vi "SimpleLiveAppStreamSaving.vi"() -> ()   [LabVIEW 2020]
uses:
  C:/Users/Public/Documents/Photometrics/PMQI-LabViewSamples/Examples/2018/Dependencies/PVCamNET.dll
  Dependencies/PVCamNET.dll
panel:
  out "Multi Page TIFF Size Read":u64 max=1 step=1
  in  "Multi Page TIFF Size [bytes]":u64 max=1 step=1
  out "Big TIFF":bool
  in  "BigTIFF On/Off":bool
  out "Available Ram":u64
  out "Disk Stream Queue Size":u64
  out "Dropped Frames":i32
  out "Buffer Index":i32
  in  "Path":path
  out "StreamSavingPath":string
  in  "File format":u8 max=1 step=1
  out "Stream Saving":bool
  out "Display":bool
  in  "Stream Saving On/Off":bool
  in  "Display On/Off":bool
  in  "Exposure Time [ms]":dbl
  in  "Live":bool
  in  "Camera Status":bool
  in  "Uninit":bool
  in  "Live stop":bool
  in  "Live start":bool
  in  "Init":bool
  # "SimpleLiveAppStreamSaving.vi\n\nDescription:\nThis sample code lets the user use stream saving with live mode in an event driven structure.\n\nSteps to run:\n1. Click \"Run\"\n2. Click \"Open\"\n3. Enter Exposure Time\n4. Turn On/Off display\n5. Set \"0\" to Format ( Raw=0 Tiff =1)\n6. Toggle Big TIFF\n7. Enter multi page TIFF size (at default the staxk size is 2GB for regular TIFF and 4GB for Big TIFF)\n8. Select the path for images to be saved at\n9. Turn \"On\" Stream Saving\n10. Click \"Live start\"\n11. Click \"Live stop\"\n12. Click \"Close\""
  # "Note about Tiff and BigTiff saving:\n\n\tAt default images are stored with regular Tiff and the maximum multi-image size is 2GB.\n\nIf you would like to save 6GB with Big Tiff then\n    BIG TIFF ON /OFF = ON;\n    Multi Page TIFF Size = 6442450944; (in bytes)\n\t\t\nIfyou would like to save 1 page per file with regular Tiff\n    BIG TIFF ON /OFF = ON;\n    Multi Page TIFF Size =1; (any number smaller than a frame size except 0)\n\t\t\nIf you would like to save 2GB with regular Tiff then\n    BIG TIFF ON /OFF = OFF;\n    Multi Page TIFF Size = 2147483648;"
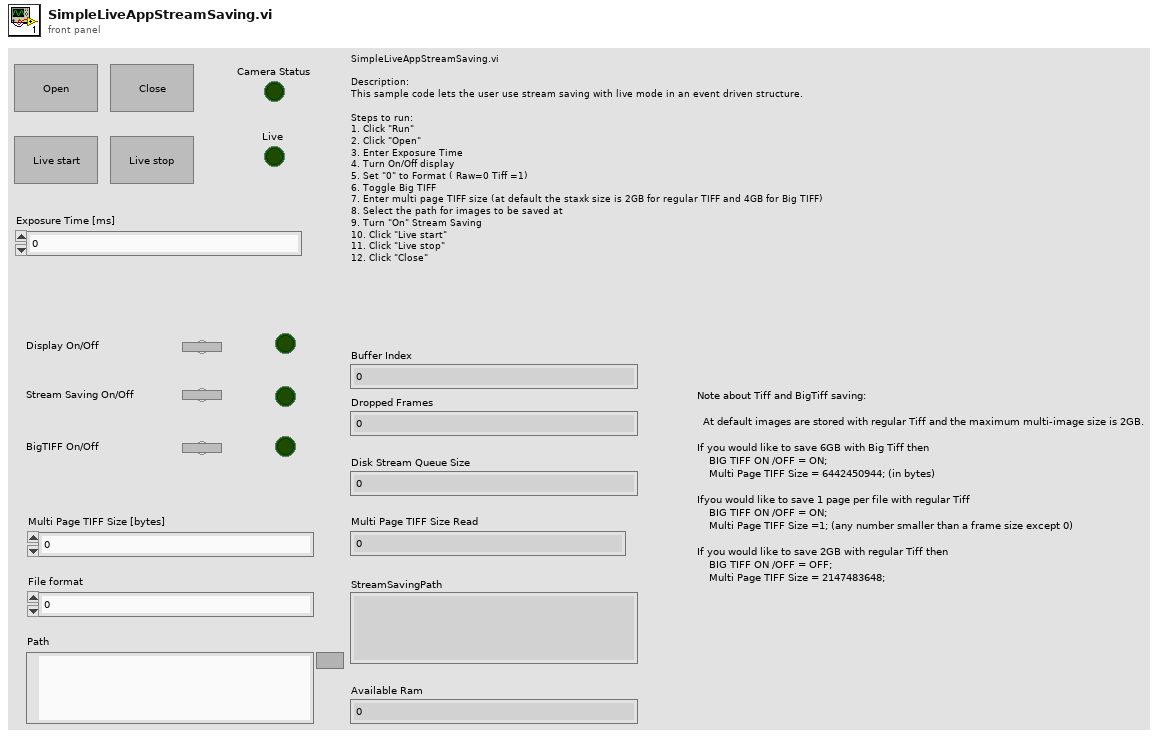
[diagram p1: front panel]
types:
  T1 = cluster{"Buffer Index":refnum<vi>, "Dropped Frames":refnum<vi>, "Disk Stream Queue Size":refnum<vi>, "Available Ram":refnum<vi>}
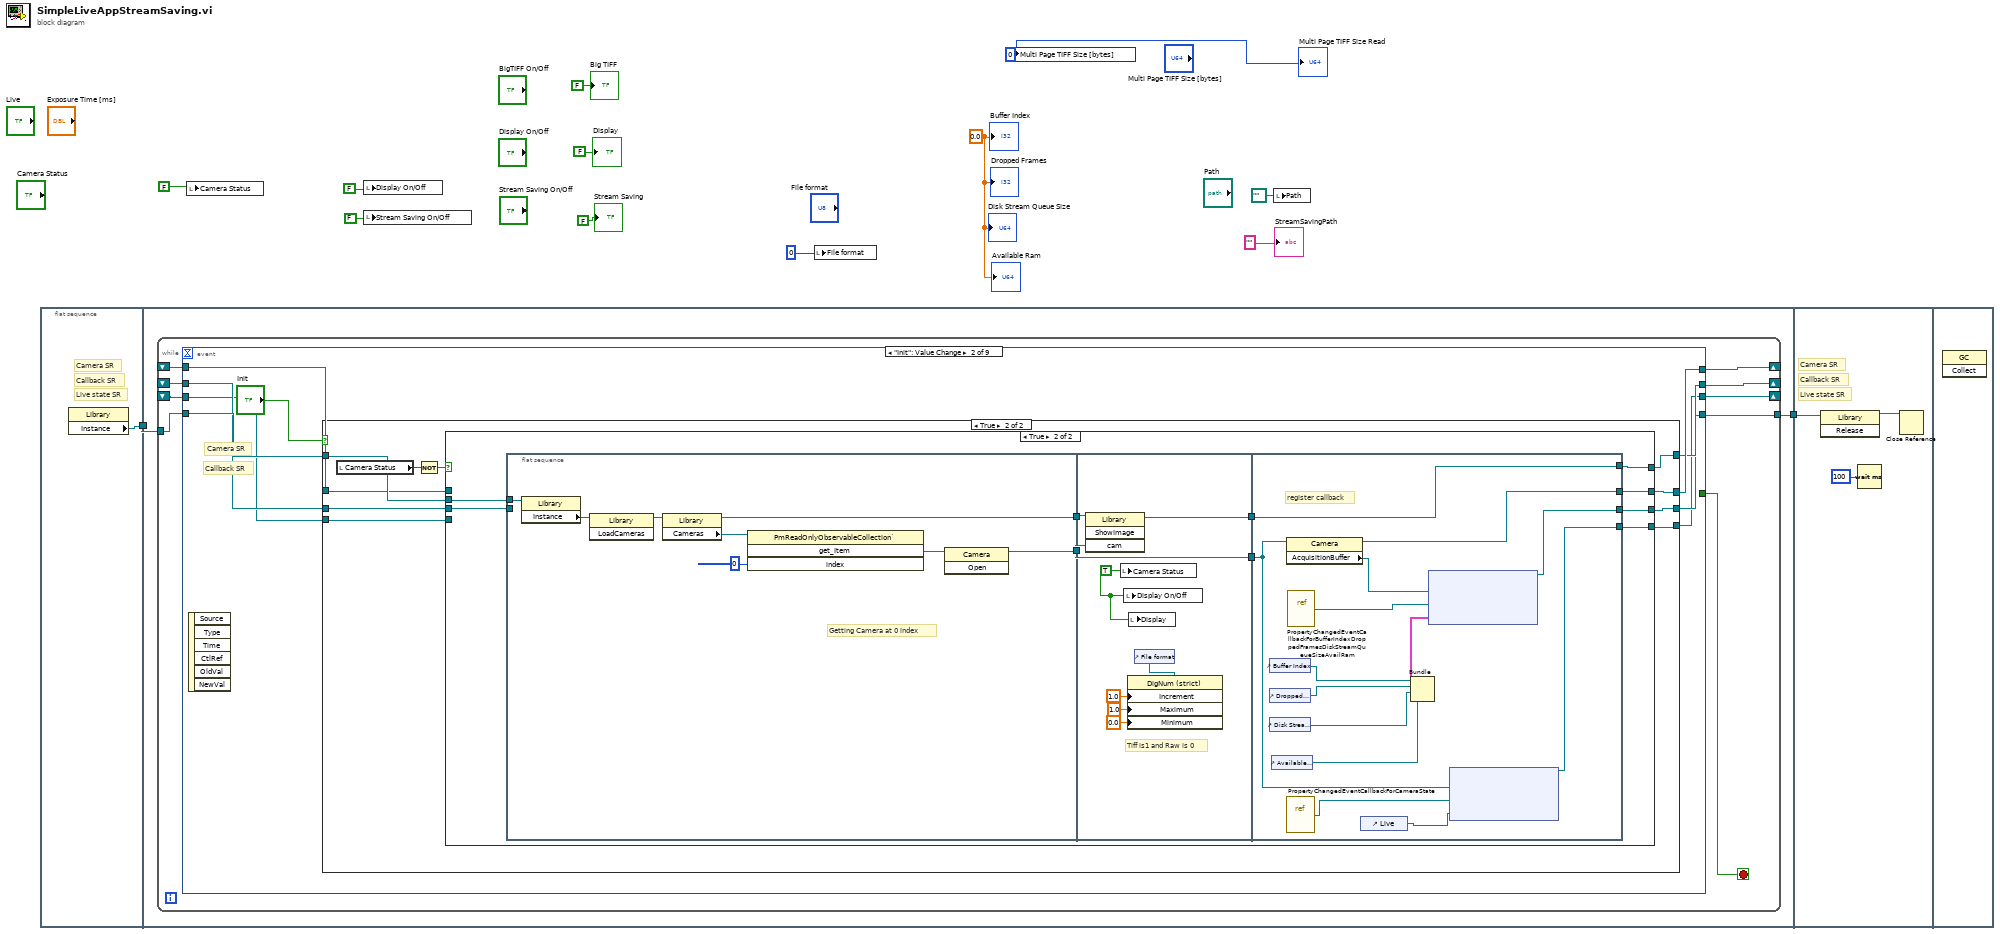
[diagram p0: block diagram]
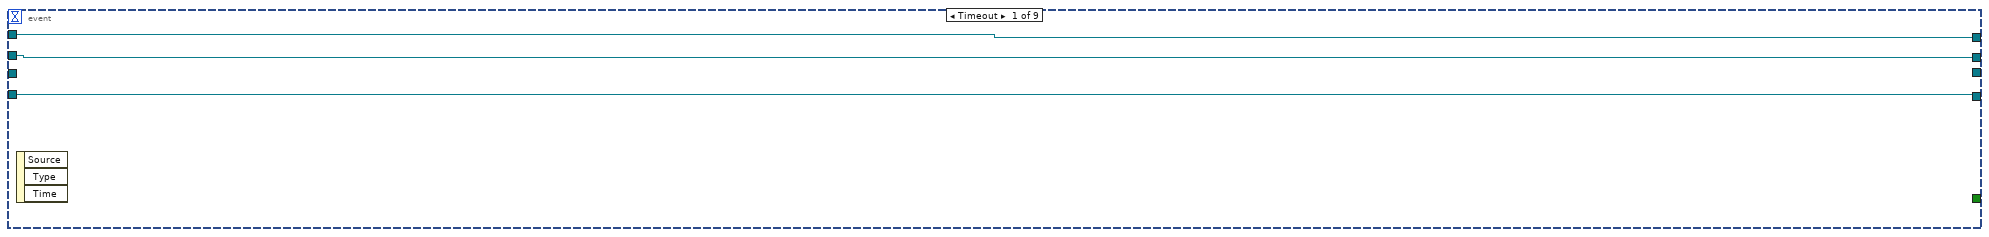
[diagram p2: hidden frame]
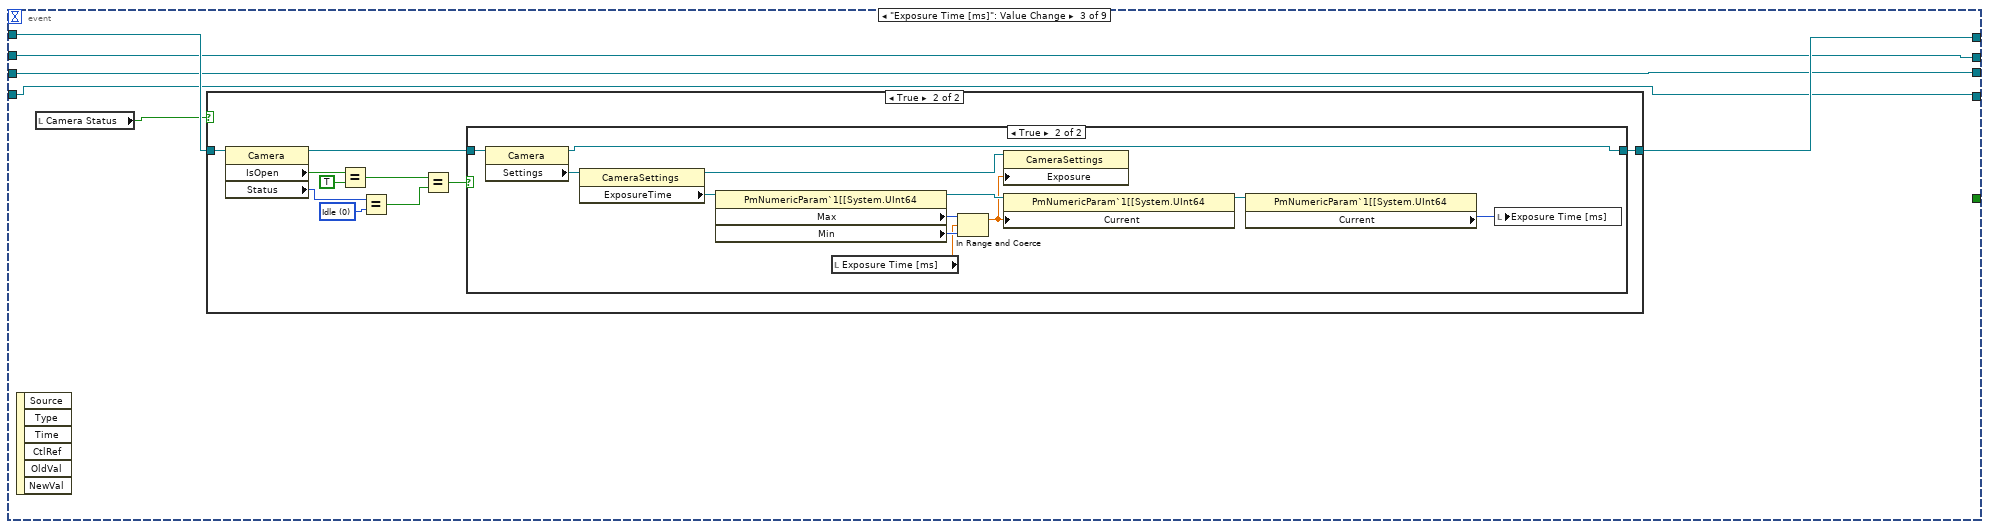
[diagram p5: hidden frame]
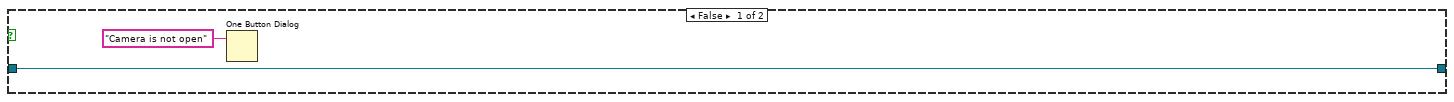
[diagram p6: hidden frame]
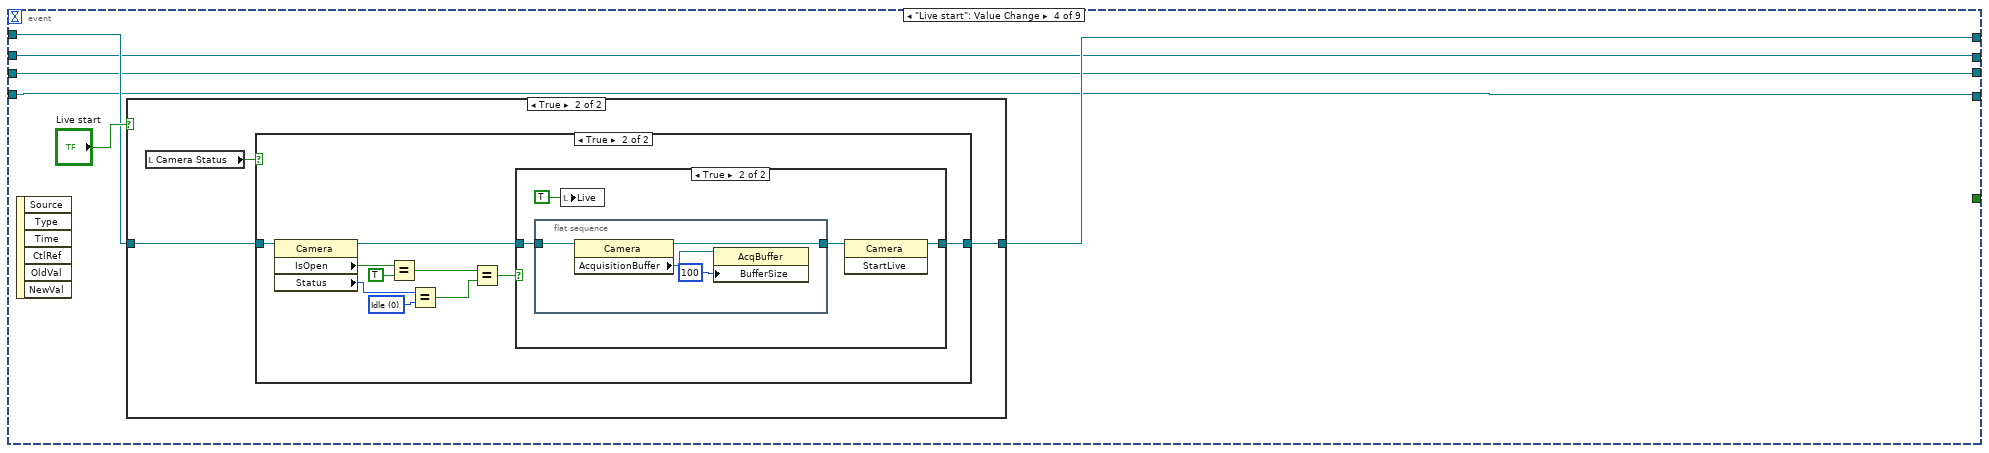
[diagram p8: hidden frame]
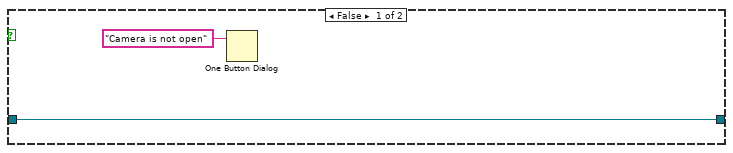
[diagram p10: hidden frame]
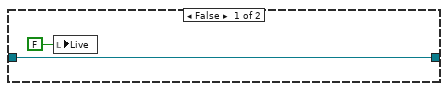
[diagram p11: hidden frame]
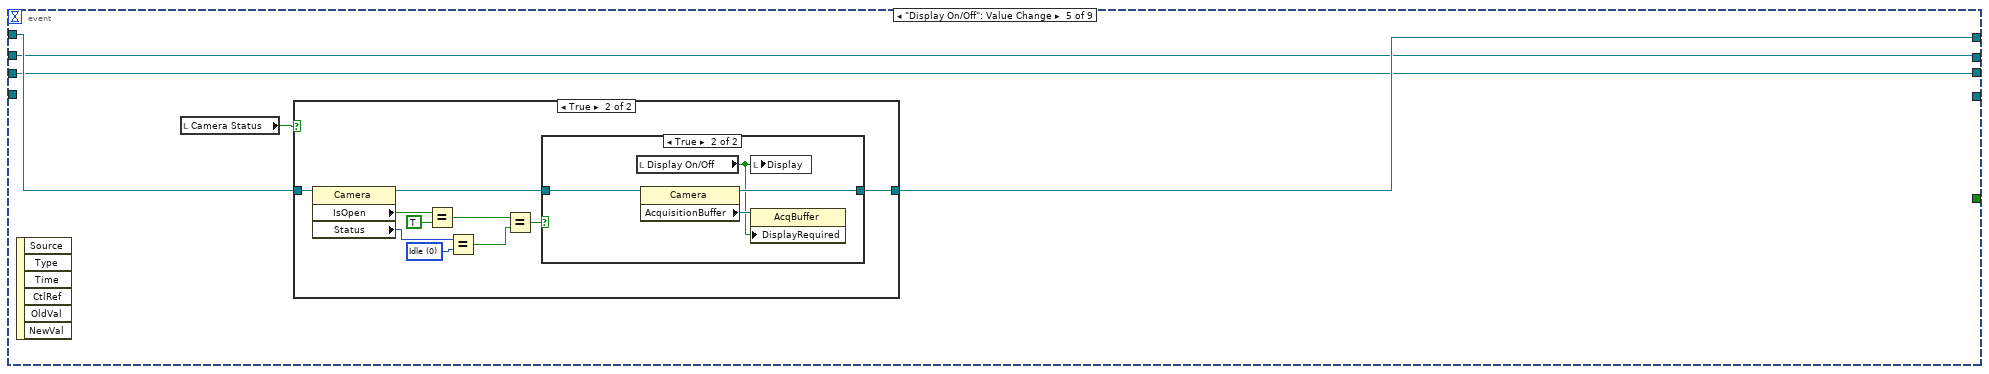
[diagram p12: hidden frame]
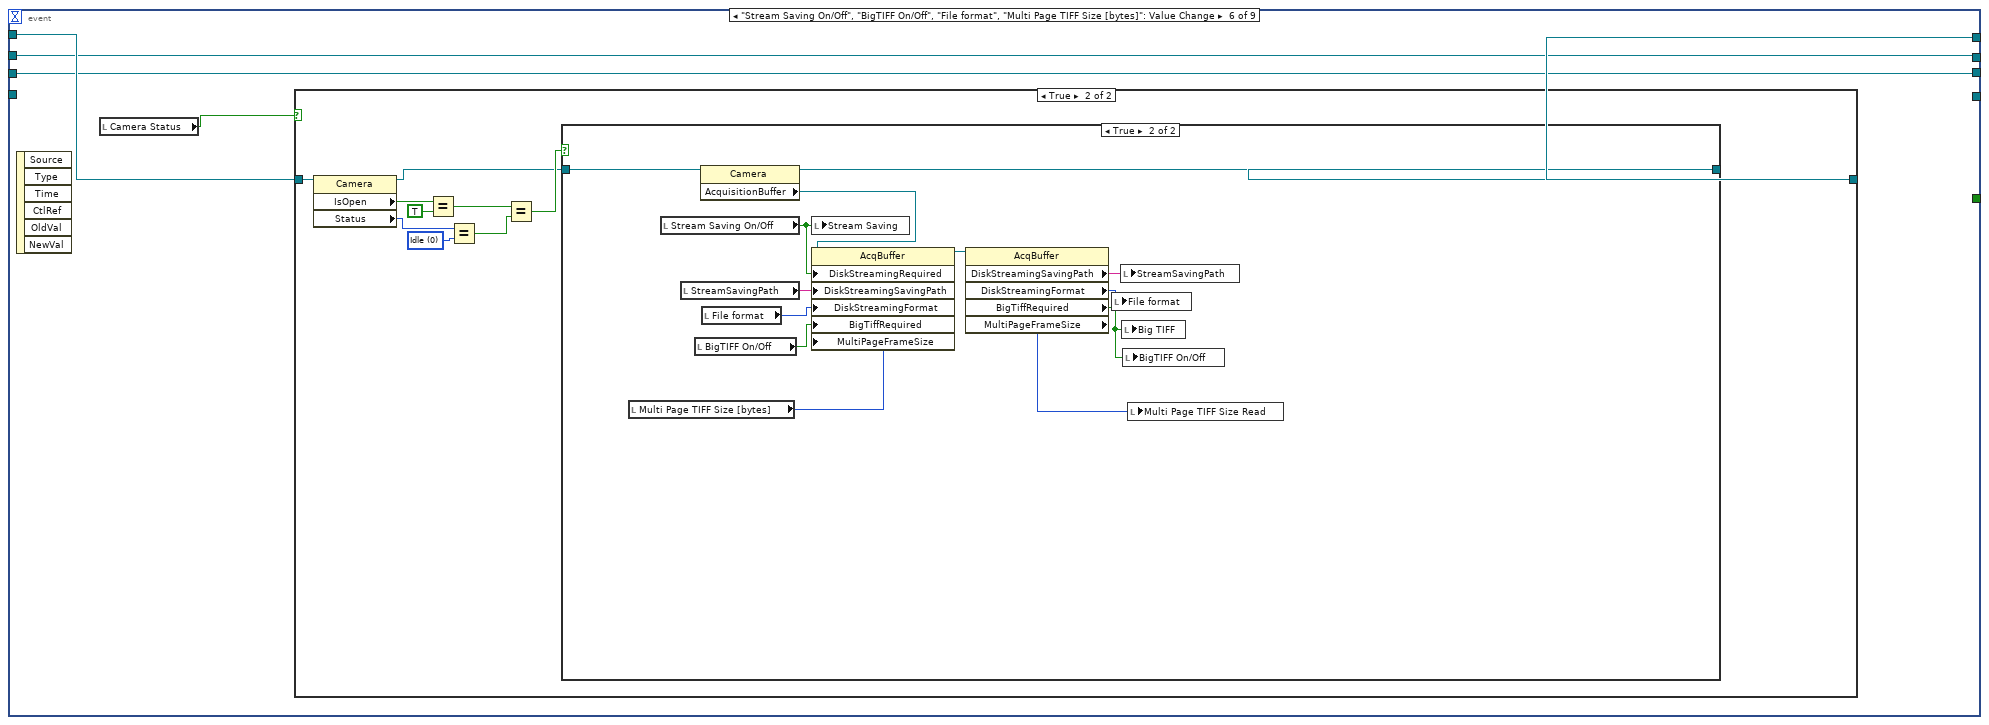
[diagram p15: hidden frame]
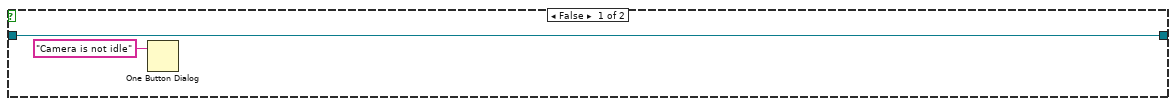
[diagram p17: hidden frame]
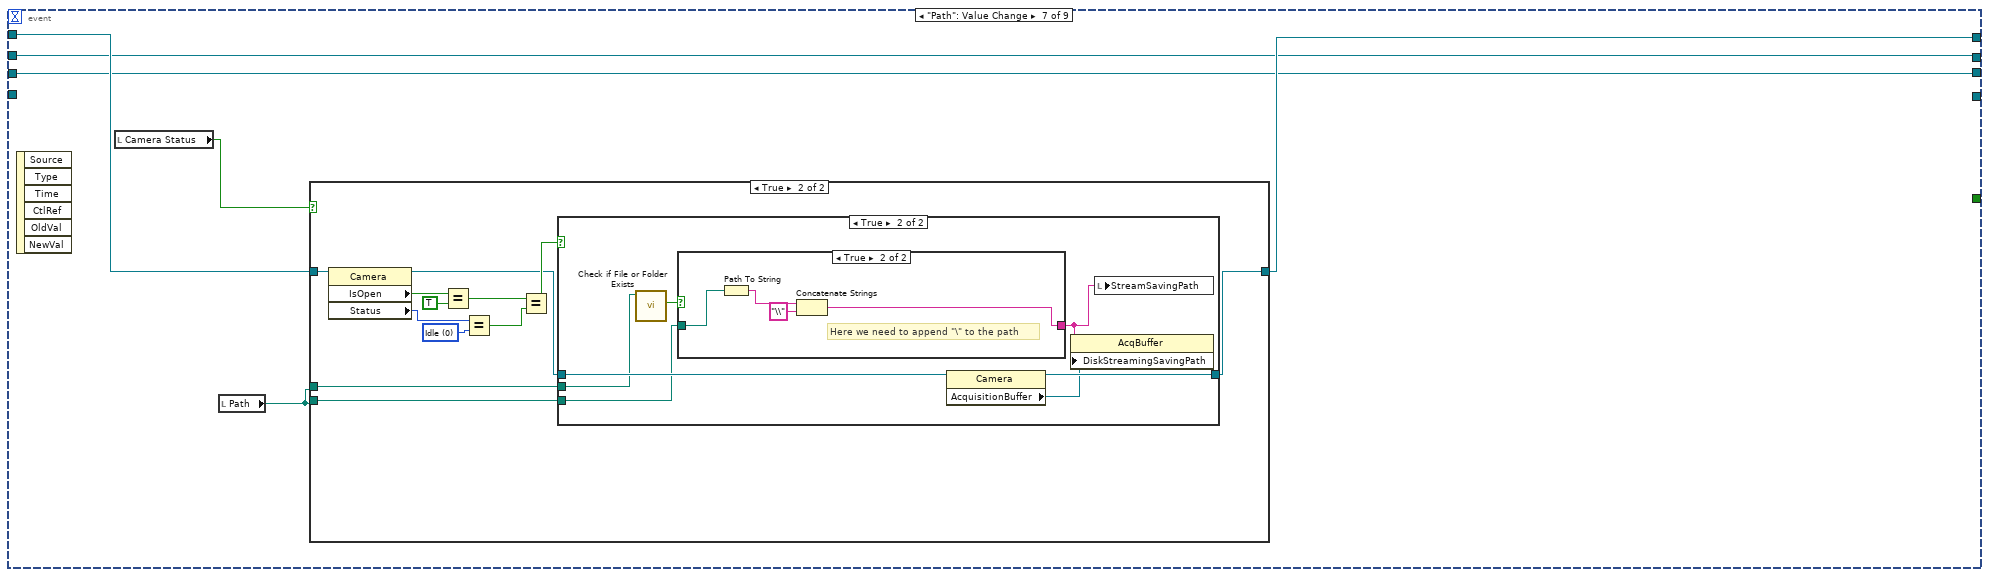
[diagram p18: hidden frame]
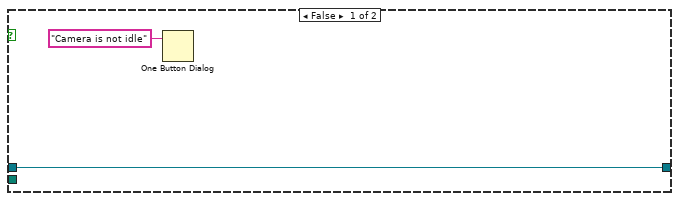
[diagram p20: hidden frame]
diagram:
  w1 = u8 0 ("Multi Page Tiff Size")
  w3 = 0.0 ("Buffer Index")
  n1 = flat-sequence {
    tunnel: [w14] -> w13
    tunnel: w13 -> [w16]
    tunnel: [w15] -> w12
    tunnel: w12 -> [w327]
    frame #0 {
      # "Live state SR"
      # "Callback SR"
      # "Camera SR"
      n2 = property class="Library"() -> ("Instance"=w14:refnum<k24>)  [unwired: 2 in, 2 out]
    }
    frame #1 {
      n3 = while {
        tunnel: w16 -> [w25]
        shift-right: [w24] -> _
        shift-left: _ -> [w22]
        tunnel: [w23] -> w15
        shift-right: [w20] -> _
        shift-left: _ -> [w19]
        shift-right: [w18] -> _
        shift-left: _ -> [w17]
        stop <- w21 stop-if-true
        n4 = event shown="[1] \"Init\": Value Change" {
          selector: _ -> [_ _ _ _ _ _ _ _ _]
          dyn-events: _ -> [_ _ _ _ _ _ _ _ _]
          timeout: _ -> [_ _ _ _ _ _ _ _ _]
          tunnel: w25 -> [w26 w37 w98 w129 _ _ _ _ w277]
          tunnel: [w27 w36 w100 w130 w162 w182 w214 w248 w278] -> w24
          tunnel: [w26 w35 w98 w129 _ _ _ _ w277] -> w23
          tunnel: w22 -> [w27 w34 w101 w131 w163 w183 w215 w249 w272]
          tunnel: [_ _ _ _ _ _ _ _ w276] -> w21
          tunnel: [w28 w32 w97 w127 w160 w181 w213 w247 w273] -> w20
          tunnel: w19 -> [w28 w31 w97 w127 w160 w181 w213 w247 w274]
          tunnel: [_ w30 w96 w128 w159 w180 w212 w245 w271] -> w18
          tunnel: w17 -> [_ w29 w96 w128 w159 w180 w212 w245 w270]
          event Timeout {
            n5 = event-data() -> ()  [unwired: 1 in, 3 out]
          }
          event "Init": Value Change {
            # "Camera SR"
            # "Callback SR"
            n6 = event-data() -> ()  [unwired: 1 in, 6 out]
            n7 = case shown="True" "Init" {
              tunnel: w37 -> [w41 w51]
              tunnel: [w40 w50] -> w36
              tunnel: [w41 w44] -> w35
              tunnel: w34 -> [w40 w47]
              tunnel: [w39 w45] -> w32
              tunnel: w31 -> [w39 w46]
              tunnel: [w38 w43] -> w30
              tunnel: w29 -> [w38 w42]
              frame False {
              }
              frame True {
                n8 = local read "Camera Status"() -> (w49:bool)
                n9 = Not(x=w49) -> (.not. x?=w48:bool)
                n10 = case shown="True" w48 {
                  tunnel: w51 -> [w54 w63]
                  tunnel: [w55 w62] -> w50
                  tunnel: [w54 w61] -> w44
                  tunnel: w47 -> [w55 _]
                  tunnel: [w53 w58] -> w45
                  tunnel: w46 -> [w53 w57]
                  tunnel: [w52 w56] -> w43
                  tunnel: w42 -> [w52 _]
                  frame False {
                  }
                  frame True {
                    n11 = flat-sequence {
                      tunnel: w63 -> [w68]
                      tunnel: [w70] -> w65
                      tunnel: [w69] -> w64
                      tunnel: w57 -> [_]
                      tunnel: w65 -> [w80]
                      tunnel: w64 -> [w81]
                      tunnel: [w81] -> w60
                      tunnel: [w79] -> w59
                      tunnel: [w95] -> w61
                      tunnel: [w89] -> w62
                      tunnel: w60 -> [w88]
                      tunnel: w59 -> [w95]
                      tunnel: [w84] -> w58
                      tunnel: [w85] -> w56
                      frame #0 {
                        # "Getting Camera at 0 index"
                        n12 = property class="Library"(reference=w68) -> ("Instance"=w67:refnum<k24>)  [unwired: 1 in, 2 out]
                        n13 = invoke class="Library" method="LoadCameras"(reference=w67) -> (reference out=w66:refnum<k24>)  [unwired: 2 in, 2 out]
                        n14 = property class="Library"(reference=w66) -> (reference out=w70:refnum<k24>, "Cameras"=w73:refnum<k24>)  [unwired: 1 in, 1 out]
                        n15 = invoke class="PmReadOnlyObservableCollection`" method="get_Item"(reference=w73, "index"=0) -> ("get_Item"=w71:refnum<k24>)  [unwired: 2 in, 3 out]
                        n16 = invoke class="Camera" method="Open"(reference=w71) -> (reference out=w69:refnum<k24>)  [unwired: 2 in, 2 out]
                      }
                      frame #1 {
                        w78 = TRUE ("Camera Status")
                        # "Tiff is1 and Raw is 0"
                        n17 = invoke class="Library" method="ShowImage"(reference=w80, "cam"=w81) -> (reference out=w79:refnum<k24>)  [unwired: 2 in, 3 out]
                        n18 = local write "Camera Status"(w78) -> ()
                        n19 = local write "Display On/Off"(w78) -> ()
                        n20 = local write "Display"(w78) -> ()
                        n21 = control-ref of="File format"() -> (w77:refnum<vi>)
                        n22 = property class="DigNum (strict)"(reference=w77, "Increment"=1.0 ("Data Entry Limits:Increment"), "Maximum"=1.0 ("Data Entry Limits:Maximum"), "Minimum"=0.0 ("Data Entry Limits:Minimum")) -> ()  [unwired: 1 in, 2 out]
                      }
                      frame #2 {
                        # "register callback"
                        n23 = control-ref of="Buffer Index"() -> (w94:refnum<vi>)
                        n24 = control-ref of="Dropped Frames"() -> (w93:refnum<vi>)
                        n25 = control-ref of="Disk Stream Queue Size"() -> (w92:refnum<vi>)
                        n26 = control-ref of="Available Ram"() -> (w83:refnum<vi>)
                        n27 = property class="Camera"(reference=w88) -> (reference out=w89:refnum<k24>, "AcquisitionBuffer"=w90:refnum<k24>)  [unwired: 1 in, 1 out]
                        n28 = vi-ref "PropertyChangedEventCallbackForCameraState.vi"() -> ("vi reference"=w87:refnum<vi>)
                        n29 = vi-ref "PropertyChangedEventCallbackForBufferIndexDroppedFramesDiskStreamQueueSizeAvailRam.vi"() -> ("vi reference"=w82:refnum<vi>)
                        n30 = control-ref of="Live"() -> (w86:refnum<vi>)
                        n31 = Bundle("Buffer Index"=w94, "Dropped Frames"=w93, "Disk Stream Queue Size"=w92, "Available Ram"=w83) -> (w91:T1)  [unwired: 1 in]
                        n32 = node(w90, w82, w91) -> (w84:refnum<k27>)  [unwired: 2 in, 1 out]
                        n33 = node(w88, w87, w86) -> (w85:refnum<k27>)  [unwired: 2 in, 1 out]
                      }
                    }
                  }
                }
              }
            }
          }
          event "Exposure Time [ms]": Value Change {
            n34 = event-data() -> ()  [unwired: 1 in, 6 out]
            n35 = local read "Camera Status"() -> (w99:bool)
            n36 = case shown="True" w99 {
              tunnel: w101 -> [w103 w107]
              tunnel: [w103 w104] -> w100
              frame False {
                n37 = One Button Dialog(message="Camera is not open") -> ()  [unwired: 1 in, 1 out]
              }
              frame True {
                w112 = 0 items=["Idle", "Capturing"] ("Status")
                n38 = property class="Camera"(reference=w107) -> (reference out=w105:refnum<k24>, "IsOpen"=w111:bool, "Status"=w113:i32)  [unwired: 1 in, 1 out]
                n39 = Equal?(x=w111, y=TRUE) -> (x = y?=w109:bool)
                n40 = Equal?(x=w113, y=w112) -> (x = y?=w108:bool)
                n41 = Equal?(x=w109, y=w108) -> (x = y?=w106:bool)
                n42 = case shown="True" w106 {
                  tunnel: w105 -> [w114 w126]
                  tunnel: [w114 w115] -> w104
                  frame False {
                  }
                  frame True {
                    n43 = property class="Camera"(reference=w126) -> (reference out=w115:refnum<k24>, "Settings"=w125:refnum<k24>)  [unwired: 1 in, 1 out]
                    n44 = property class="CameraSettings"(reference=w125) -> (reference out=w118:refnum<k24>, "ExposureTime"=w119:refnum<k24>)  [unwired: 1 in, 1 out]
                    n45 = property class="PmNumericParam`1[[System.UInt64"(reference=w119) -> (reference out=w122:refnum<k24>, "Max"=w124:u64, "Min"=w123:u64)  [unwired: 1 in, 1 out]
                    n46 = local read "Exposure Time [ms]"() -> (w117:dbl)
                    n47 = In Range and Coerce(upper limit=w124, x=w117, lower limit=w123) -> (coerced(x)=w120:dbl)  [unwired: 1 out]
                    n48 = property class="CameraSettings"(reference=w118, "Exposure"=w120) -> ()  [unwired: 1 in, 2 out]
                    n49 = property class="PmNumericParam`1[[System.UInt64"(reference=w122, "Current"=w120) -> (reference out=w121:refnum<k24>)  [unwired: 1 in, 1 out]
                    n50 = property class="PmNumericParam`1[[System.UInt64"(reference=w121) -> ("Current"=w116:u64)  [unwired: 1 in, 2 out]
                    n51 = local write "Exposure Time [ms]"(w116) -> ()
                  }
                }
              }
            }
          }
          event "Live start": Value Change {
            n52 = event-data() -> ()  [unwired: 1 in, 6 out]
            n53 = case shown="True" "Live start" {
              tunnel: w131 -> [w133 w136]
              tunnel: [w133 w135] -> w130
              frame False {
              }
              frame True {
                n54 = local read "Camera Status"() -> (w134:bool)
                n55 = case shown="True" w134 {
                  tunnel: w136 -> [w137 w142]
                  tunnel: [w137 w140] -> w135
                  frame False {
                    n56 = One Button Dialog(message="Camera is not open") -> ()  [unwired: 1 in, 1 out]
                  }
                  frame True {
                    w147 = 0 items=["Idle", "Capturing"] ("Status")
                    n57 = property class="Camera"(reference=w142) -> (reference out=w141:refnum<k24>, "IsOpen"=w146:bool, "Status"=w148:i32)  [unwired: 1 in, 1 out]
                    n58 = Equal?(x=w146, y=TRUE) -> (x = y?=w144:bool)
                    n59 = Equal?(x=w148, y=w147) -> (x = y?=w143:bool)
                    n60 = Equal?(x=w144, y=w143) -> (x = y?=w139:bool)
                    n61 = case shown="True" w139 {
                      tunnel: w141 -> [w150 w152]
                      tunnel: [w150 w153] -> w140
                      frame False {
                        n62 = local write "Live"(FALSE ("Live 2")) -> ()
                      }
                      frame True {
                        n63 = flat-sequence {
                          tunnel: w152 -> [w158]
                          tunnel: [w155] -> w151
                          frame #0 {
                            n64 = property class="Camera"(reference=w158) -> (reference out=w155:refnum<k24>, "AcquisitionBuffer"=w157:refnum<k24>)  [unwired: 1 in, 1 out]
                            n65 = property class="AcqBuffer"(reference=w157, "BufferSize"=100) -> ()  [unwired: 1 in, 2 out]
                          }
                        }
                        n66 = local write "Live"(TRUE ("Live")) -> ()
                        n67 = invoke class="Camera" method="StartLive"(reference=w151) -> (reference out=w153:refnum<k24>)  [unwired: 2 in, 2 out]
                      }
                    }
                  }
                }
              }
            }
          }
          event "Display On/Off": Value Change {
            n68 = event-data() -> ()  [unwired: 1 in, 6 out]
            n69 = local read "Camera Status"() -> (w161:bool)
            n70 = case shown="True" w161 {
              tunnel: w163 -> [w164 w168]
              tunnel: [w164 w165] -> w162
              frame False {
              }
              frame True {
                w173 = 0 items=["Idle", "Capturing"] ("Status")
                n71 = property class="Camera"(reference=w168) -> (reference out=w166:refnum<k24>, "IsOpen"=w172:bool, "Status"=w174:i32)  [unwired: 1 in, 1 out]
                n72 = Equal?(x=w172, y=TRUE) -> (x = y?=w170:bool)
                n73 = Equal?(x=w174, y=w173) -> (x = y?=w169:bool)
                n74 = Equal?(x=w170, y=w169) -> (x = y?=w167:bool)
                n75 = case shown="True" w167 {
                  tunnel: w166 -> [w175 w179]
                  tunnel: [w175 w177] -> w165
                  frame False {
                  }
                  frame True {
                    n76 = local read "Display On/Off"() -> (w176:bool)
                    n77 = property class="Camera"(reference=w179) -> (reference out=w177:refnum<k24>, "AcquisitionBuffer"=w178:refnum<k24>)  [unwired: 1 in, 1 out]
                    n78 = local write "Display"(w176) -> ()
                    n79 = property class="AcqBuffer"(reference=w178, "DisplayRequired"=w176) -> ()  [unwired: 1 in, 2 out]
                  }
                }
              }
            }
          }
          event "Stream Saving On/Off", "BigTIFF On/Off", "File format", "Multi Page TIFF Size [bytes]": Value Change {
            n80 = event-data() -> ()  [unwired: 1 in, 6 out]
            n81 = local read "Camera Status"() -> (w184:bool)
            n82 = case shown="True" w184 {
              tunnel: w183 -> [w185 w189]
              tunnel: [w185 w186] -> w182
              frame False {
              }
              frame True {
                w194 = 0 items=["Idle", "Capturing"] ("Status")
                n83 = property class="Camera"(reference=w189) -> (reference out=w187:refnum<k24>, "IsOpen"=w193:bool, "Status"=w195:i32)  [unwired: 1 in, 1 out]
                n84 = Equal?(x=w193, y=TRUE) -> (x = y?=w191:bool)
                n85 = Equal?(x=w195, y=w194) -> (x = y?=w190:bool)
                n86 = Equal?(x=w191, y=w190) -> (x = y?=w188:bool)
                n87 = case shown="True" w188 {
                  tunnel: w187 -> [w197 w210]
                  tunnel: [w197 w209] -> w186
                  frame False {
                    n88 = One Button Dialog(message="Camera is not idle") -> ()  [unwired: 1 in, 1 out]
                  }
                  frame True {
                    n89 = local read "Multi Page TIFF Size [bytes]"() -> (w199:u64)
                    n90 = local read "Stream Saving On/Off"() -> (w207:bool)
                    n91 = local read "StreamSavingPath"() -> (w206:string)
                    n92 = local read "BigTIFF On/Off"() -> (w200:bool)
                    n93 = property class="Camera"(reference=w210) -> (reference out=w209:refnum<k24>, "AcquisitionBuffer"=w208:refnum<k24>)  [unwired: 1 in, 1 out]
                    n94 = local read "File format"() -> (w205:u8)
                    n95 = local write "Stream Saving"(w207) -> ()
                    n96 = property class="AcqBuffer"(reference=w208, "DiskStreamingRequired"=w207, "DiskStreamingSavingPath"=w206, "DiskStreamingFormat"=w205, "BigTiffRequired"=w200, "MultiPageFrameSize"=w199) -> (reference out=w202:refnum<k24>)  [unwired: 1 in, 1 out]
                    n97 = property class="AcqBuffer"(reference=w202) -> ("DiskStreamingSavingPath"=w203:string, "DiskStreamingFormat"=w204:u32, "BigTiffRequired"=w201:bool, "MultiPageFrameSize"=w198:u64)  [unwired: 1 in, 2 out]
                    n98 = local write "File format"(w204) -> ()
                    n99 = local write "StreamSavingPath"(w203) -> ()
                    n100 = local write "Big TIFF"(w201) -> ()
                    n101 = local write "BigTIFF On/Off"(w201) -> ()
                    n102 = local write "Multi Page TIFF Size Read"(w198) -> ()
                  }
                }
              }
            }
          }
          event "Path": Value Change {
            n103 = event-data() -> ()  [unwired: 1 in, 6 out]
            n104 = local read "Camera Status"() -> (w216:bool)
            n105 = local read "Path"() -> (w211:path)
            n106 = case shown="True" w216 {
              tunnel: w215 -> [w217 w223]
              tunnel: [w217 w220] -> w214
              tunnel: w211 -> [_ w219]
              tunnel: w211 -> [_ w218]
              frame False {
              }
              frame True {
                w228 = 0 items=["Idle", "Capturing"] ("Status")
                n107 = property class="Camera"(reference=w223) -> (reference out=w221:refnum<k24>, "IsOpen"=w227:bool, "Status"=w229:i32)  [unwired: 1 in, 1 out]
                n108 = Equal?(x=w227, y=TRUE) -> (x = y?=w225:bool)
                n109 = Equal?(x=w229, y=w228) -> (x = y?=w224:bool)
                n110 = Equal?(x=w225, y=w224) -> (x = y?=w222:bool)
                n111 = case shown="True" w222 {
                  tunnel: w221 -> [w231 w238]
                  tunnel: [w231 w237] -> w220
                  tunnel: w219 -> [_ w234]
                  tunnel: w218 -> [_ w233]
                  frame False {
                    n112 = One Button Dialog(message="Camera is not idle") -> ()  [unwired: 1 in, 1 out]
                  }
                  frame True {
                    n113 = call <vilib>:"Check if File or Folder Exists.vi"("path"=w233) -> ("file or folder exists?"=w235:bool)  [unwired: 8 in, 2 out]
                    n114 = case shown="True" w235 {
                      tunnel: w234 -> [_ w244]
                      tunnel: ["" w241] -> w232
                      frame False {
                        n115 = One Button Dialog(message="The specified folder doesn't exist") -> ()  [unwired: 1 in, 1 out]
                      }
                      frame True {
                        # "Here we need to append \"\\\" to the path"
                        n116 = Path To String(path=w244) -> (string=w243:string)
                        n117 = Concatenate Strings(w243, "\\" ("string")) -> (w241:string)
                      }
                    }
                    n118 = property class="Camera"(reference=w238) -> (reference out=w237:refnum<k24>, "AcquisitionBuffer"=w236:refnum<k24>)  [unwired: 1 in, 1 out]
                    n119 = property class="AcqBuffer"(reference=w236, "DiskStreamingSavingPath"=w232) -> ()  [unwired: 1 in, 2 out]
                    n120 = local write "StreamSavingPath"(w232) -> ()
                  }
                }
              }
            }
          }
          event "Live stop": Value Change {
            n121 = event-data() -> ()  [unwired: 1 in, 6 out]
            n122 = case shown="True" "Live stop" {
              tunnel: w249 -> [w250 w253]
              tunnel: [w250 w252] -> w248
              frame False {
              }
              frame True {
                n123 = local read "Camera Status"() -> (w251:bool)
                n124 = case shown="True" w251 {
                  tunnel: w253 -> [w255 w265]
                  tunnel: [w255 w262] -> w252
                  frame False {
                    n125 = One Button Dialog(message="Camera is not open") -> ()  [unwired: 1 in, 1 out]
                  }
                  frame True {
                    w260 = 1 items=["Idle", "Capturing"] ("Status")
                    n126 = property class="Camera"(reference=w265) -> (reference out=w263:refnum<k24>, "IsOpen"=w259:bool, "Status"=w261:i32)  [unwired: 1 in, 1 out]
                    n127 = Equal?(x=w261, y=w260) -> (x = y?=w256:bool)
                    n128 = Equal?(x=w259, y=TRUE) -> (x = y?=w257:bool)
                    n129 = Equal?(x=w257, y=w256) -> (x = y?=w264:bool)
                    n130 = case shown="True" w264 {
                      tunnel: w263 -> [w266 w269]
                      tunnel: [w266 w268] -> w262
                      frame False {
                      }
                      frame True {
                        n131 = invoke class="Camera" method="Stop"(reference=w269) -> (reference out=w268:refnum<k24>)  [unwired: 2 in, 2 out]
                        n132 = local write "Live"(FALSE ("Live 2")) -> ()
                      }
                    }
                  }
                }
              }
            }
          }
          event "Uninit": Value Change {
            n133 = event-data() -> ()  [unwired: 1 in, 6 out]
            n134 = case shown="True" "Uninit" {
              tunnel: w272 -> [w282 w290]
              tunnel: [w282 w289] -> w278
              tunnel: [FALSE ("Camera Status") w287] -> w276
              tunnel: w274 -> [w280 w286]
              tunnel: [w280 w285] -> w273
              tunnel: [w279 w284] -> w271
              tunnel: w270 -> [w279 w283]
              frame False {
              }
              frame True {
                n135 = local read "Camera Status"() -> (w288:bool)
                n136 = case shown="True" w288 {
                  tunnel: w290 -> [w294 w303]
                  tunnel: [w294 w302] -> w289
                  tunnel: [FALSE ("Camera Status") w301] -> w287
                  tunnel: w286 -> [w292 w298]
                  tunnel: [w292 w297] -> w285
                  tunnel: [w291 w296] -> w284
                  tunnel: w283 -> [w291 w295]
                  frame False {
                  }
                  frame True {
                    n137 = local read "Live"() -> (w299:bool)
                    n138 = Not(x=w299) -> (.not. x?=w300:bool)
                    n139 = case shown="True" w300 {
                      tunnel: w303 -> [w307 w314]
                      tunnel: [w307 w313] -> w302
                      tunnel: [FALSE ("Camera Status") w312] -> w301
                      tunnel: w298 -> [w305 w311]
                      tunnel: [w305 w310] -> w297
                      tunnel: [w304 w309] -> w296
                      tunnel: w295 -> [w304 w308]
                      frame False {
                      }
                      frame True {
                        n140 = flat-sequence {
                          tunnel: w314 -> [w319]
                          tunnel: [w318] -> w315
                          tunnel: w311 -> [w317]
                          tunnel: w308 -> [w316]
                          tunnel: [w325] -> w313
                          tunnel: w315 -> [w325]
                          tunnel: [TRUE ("Camera Status")] -> w312
                          tunnel: [refnum<k27> refnum ("Event Callback")] -> w310
                          tunnel: [refnum<k27> refnum ("Event Callback")] -> w309
                          frame #0 {
                            n141 = invoke class="Camera" method="Close"(reference=w319) -> (reference out=w318:refnum<k24>)  [unwired: 2 in, 2 out]
                            n142 = Unregister For Events(event registration refnum=w317) -> ()  [unwired: 1 in, 1 out]
                            n143 = Unregister For Events(event registration refnum=w316) -> ()  [unwired: 1 in, 1 out]
                          }
                          frame #1 {
                            w320 = FALSE ("Big TIFF On/Off")
                            n144 = local write "Camera Status"(FALSE ("Camera Status")) -> ()
                            n145 = local write "Display On/Off"(w320) -> ()
                            n146 = local write "Stream Saving On/Off"(w320) -> ()
                            n147 = local write "BigTIFF On/Off"(w320) -> ()
                            n148 = local write "Stream Saving"(w320) -> ()
                            n149 = local write "Display"(w320) -> ()
                            n150 = local write "Big TIFF"(w320) -> ()
                          }
                        }
                      }
                    }
                  }
                }
              }
            }
          }
        }
      }
    }
    frame #2 {
      # "Live state SR"
      # "Callback SR"
      # "Camera SR"
      n151 = invoke class="Library" method="Release"(reference=w327) -> (reference out=w328:refnum<k24>)  [unwired: 2 in, 2 out]
      n152 = Wait (ms)(milliseconds to wait=u32 100) -> ()  [unwired: 1 out]
      n153 = Close Reference(reference=w328) -> ()  [unwired: 1 in, 1 out]
    }
    frame #3 {
      n154 = invoke class="GC" method="Collect"() -> ()  [unwired: 3 in, 3 out]
    }
  }
  n155 = local write "Camera Status"(FALSE ("Camera Status")) -> ()
  n156 = local write "Display On/Off"(FALSE ("Raw On/Off")) -> ()
  n157 = local write "Stream Saving On/Off"(FALSE ("Raw On/Off")) -> ()
  n158 = local write "File format"(u8 0 ("Tiff==0 Raw==1")) -> ()
  n159 = local write "Multi Page TIFF Size [bytes]"(w1) -> ()
  n160 = local write "Path"(path "" ("Path")) -> ()
  "Display" <- FALSE ("Display")
  "Stream Saving" <- FALSE ("Display")
  "StreamSavingPath" <- "" ("StreamSavingPath")
  "Disk Stream Queue Size" <- w3
  "Dropped Frames" <- w3
  "Buffer Index" <- w3
  "Available Ram" <- w3
  "Big TIFF" <- FALSE ("Big TIFF")
  "Multi Page TIFF Size Read" <- w1
